vi "Sub_Online_FFT.vi"(9 "Bound to 1st Frequency":bool=TRUE, 10 "Frequency Method":T4(ring), 11 "Experiment in":T1) -> (3 "Experiment out":T2)   [LabVIEW 2021]
uses:
  Control 1.ctl
  <vilib>/Analysis/4window.llb/Hanning Window (DBL).vi
  <vilib>/Analysis/5stat.llb/RMS (DBL).vi
  <vilib>/Analysis/4window.llb/Hamming Window (DBL).vi
  <vilib>/Analysis/2dsp.llb/Real FFT.vi
  <vilib>/Analysis/4window.llb/AllCosWindow (DBL).vi
  <vilib>/addons/Time Series Analysis/Series Preprocess.llb/TSA Moving Average (Array).vi
  <vilib>/Analysis/NI_AALPro.lvlib
  <vilib>/addons/_Advanced Signal Processing/NI_AdvSigProcTSA.lvlib
panel:
  in  "Frequency selection method":T3(ring)
  in  "Use Top N freq components":i32=5 min=1 max=50 step=1
  out "Low-Energy Warning":bool
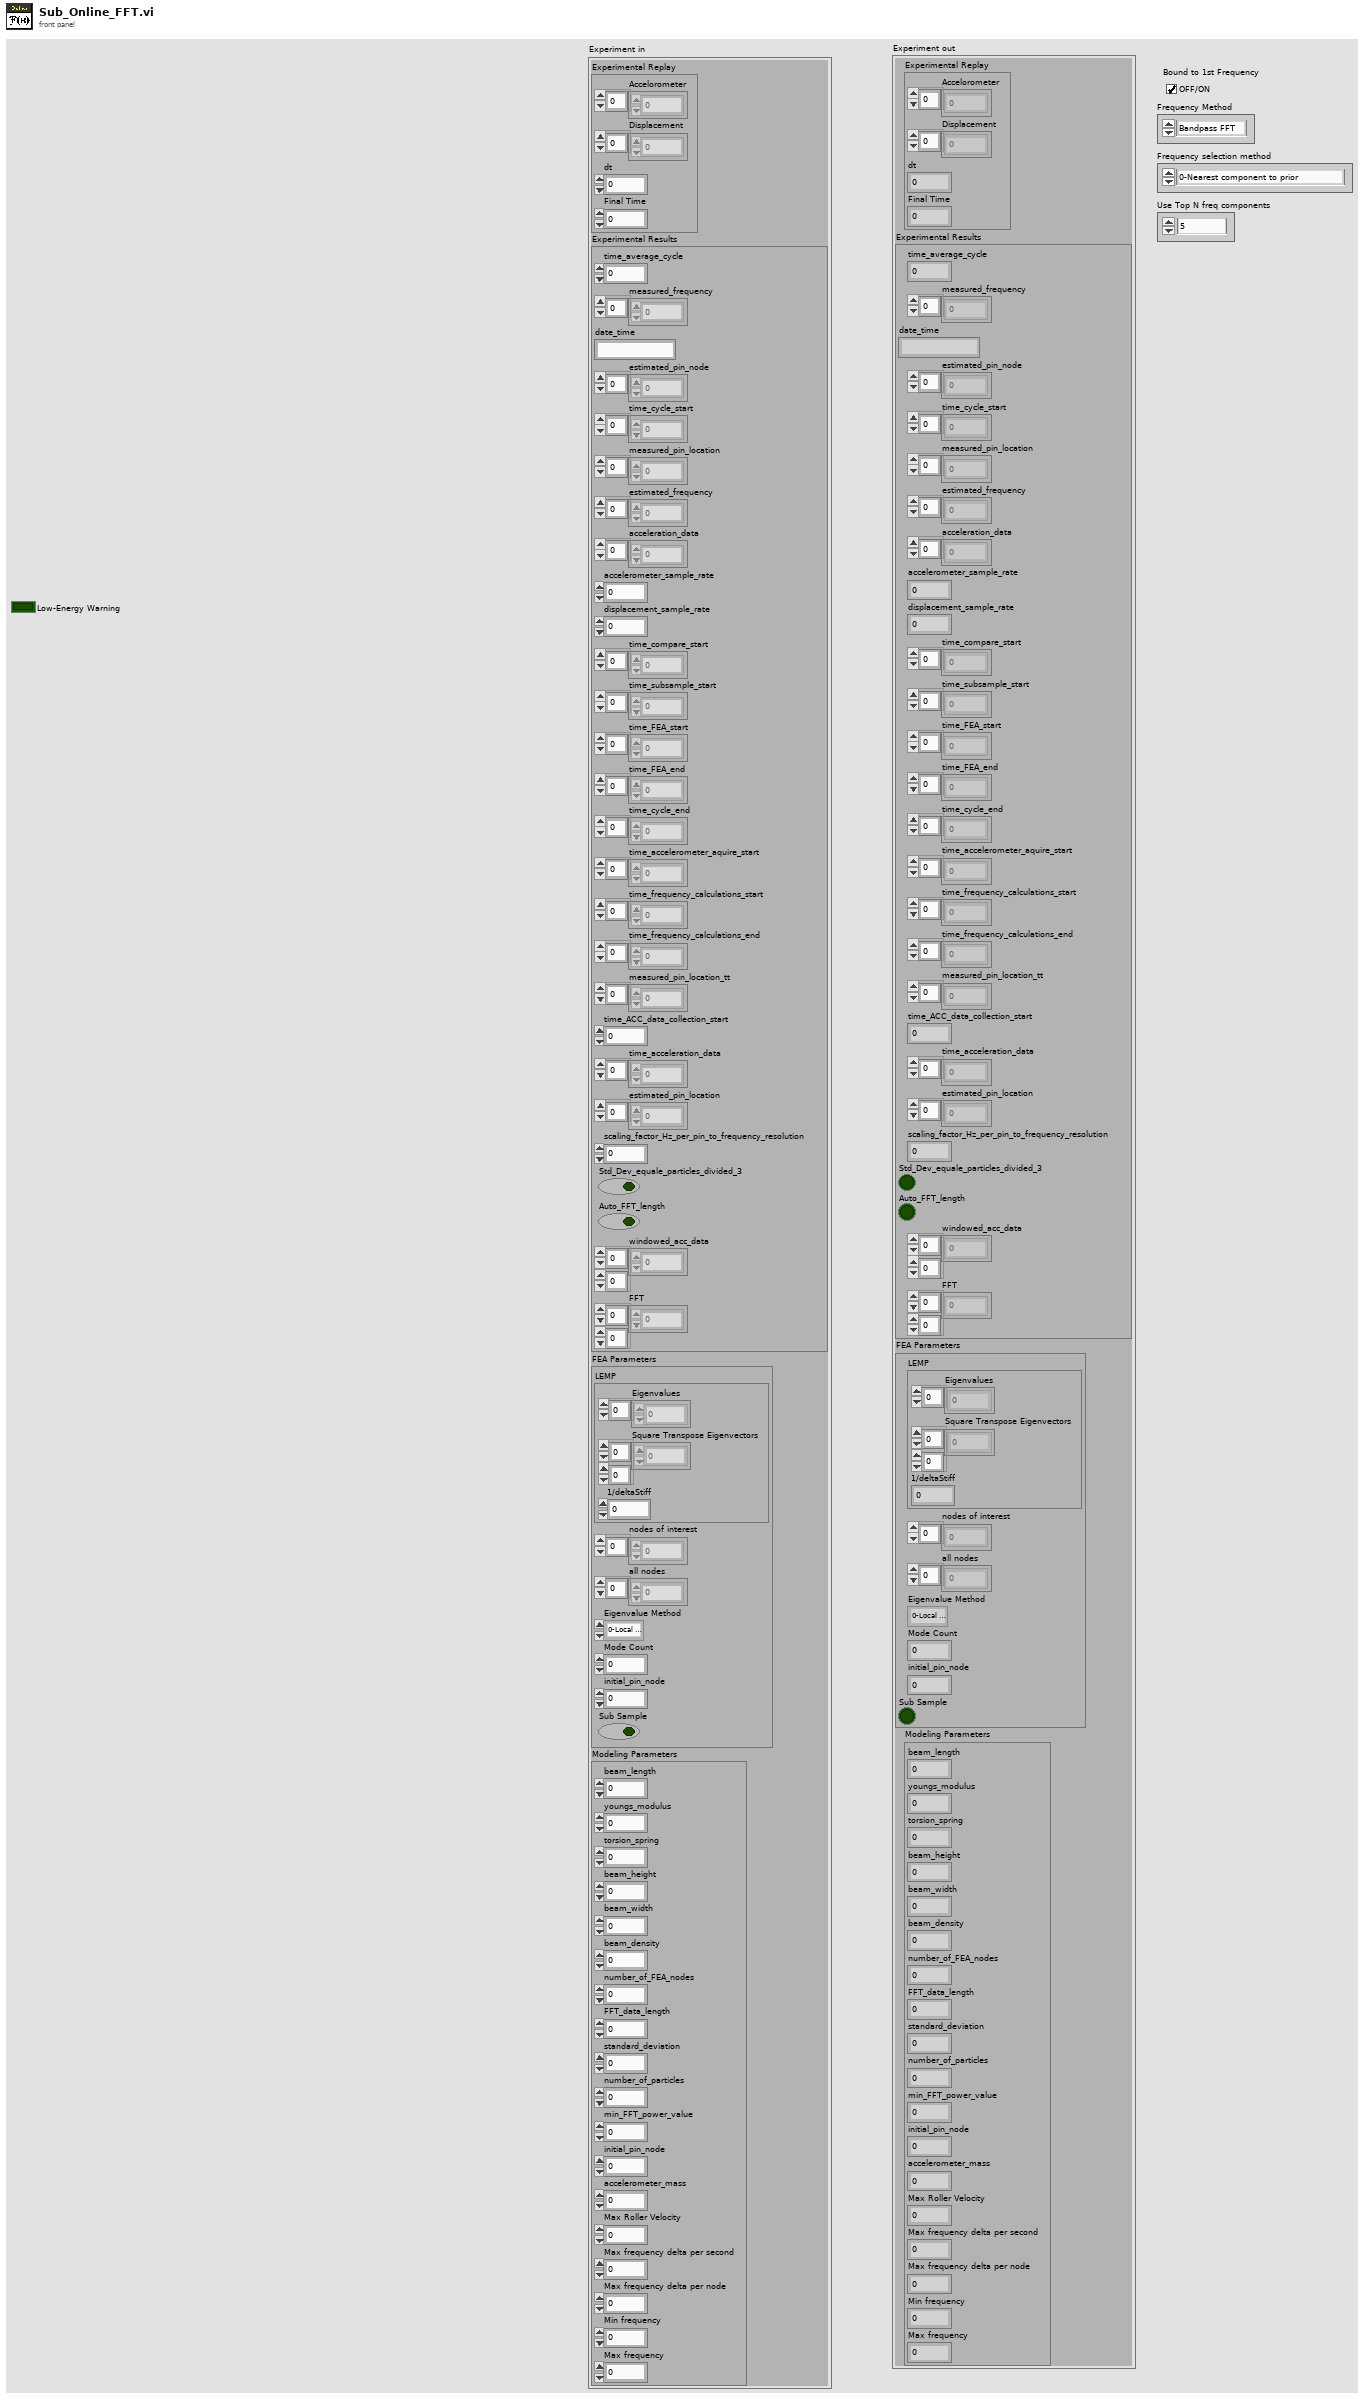
[diagram p1: front panel]
types:
  T1 = cluster{"Experimental Replay":cluster{"Accelorometer":dbl[], "Displacement":dbl[], "dt":dbl, "Final Time":dbl}, "Experimental Results":cluster{"time_average_cycle":dbl, "measured_frequency":dbl[], "date_time":string, "estimated_pin_node":i32[], "time_cycle_start":dbl[], "measured_pin_location":dbl[], "estimated_frequency":dbl[], "acceleration_data":dbl[], "accelerometer_sample_rate":dbl, "displacement_sample_rate":dbl, "time_compare_start":dbl[], "time_subsample_start":dbl[], "time_FEA_start":dbl[], "time_FEA_end":dbl[], "time_cycle_end":dbl[], "time_accelerometer_aquire_start":dbl[], "time_frequency_calculations_start":dbl[], "time_frequency_calculations_end":dbl[], "measured_pin_location_tt":dbl[], "time_ACC_data_collection_start":dbl, "time_acceleration_data":dbl[], "estimated_pin_location":dbl[], "scaling_factor_Hz_per_pin_to_frequency_resolution":dbl, "Std_Dev_equale_particles_divided_3":bool, "Auto_FFT_length":bool, "windowed_acc_data":dbl[][], "FFT":dbl[][]}, "FEA Parameters":cluster{"LEMP":cluster{"Eigenvalues":dbl[], "Square Transpose Eigenvectors":dbl[][], "1/deltaStiff":dbl}, "nodes of interest":i32[], "all nodes":i32[], "Eigenvalue Method":enum16{"0-Local Eigen Modification Procedure", "1-LabVIEW generalized eigenvalues", "2-LabVIEW M^-1K eigenvalues", "3-LabVIEW Cholesky Factorization", "4-Cholesky Factorization CPU SGL", "5-Cholesky Factorization CPU FXP", "6-Cholesky Factorization FPGA SGL", "7-Cholesky Factorization FPGA SGL SCL"}, "Mode Count":i32, "initial_pin_node":i32, "Sub Sample":bool}, "Modeling Parameters":cluster{"beam_length":dbl, "youngs_modulus":dbl, "torsion_spring":dbl, "beam_height":dbl, "beam_width":dbl, "beam_density":dbl, "number_of_FEA_nodes":i32, "FFT_data_length":i32, "standard_deviation":dbl, "number_of_particles":i32, "min_FFT_power_value":dbl, "initial_pin_node":i32, "accelerometer_mass":dbl, "Max Roller Velocity":dbl, "Max frequency delta per second":dbl, "Max frequency delta per node":dbl, "Min frequency":dbl, "Max frequency":dbl}}
  T2 = typedef "Control 1.ctl" = cluster{"Experimental Replay":cluster{"Accelorometer":dbl[], "Displacement":dbl[], "dt":dbl, "Final Time":dbl}, "Experimental Results":cluster{"time_average_cycle":dbl, "measured_frequency":dbl[], "date_time":string, "estimated_pin_node":i32[], "time_cycle_start":dbl[], "measured_pin_location":dbl[], "estimated_frequency":dbl[], "acceleration_data":dbl[], "accelerometer_sample_rate":dbl, "displacement_sample_rate":dbl, "time_compare_start":dbl[], "time_subsample_start":dbl[], "time_FEA_start":dbl[], "time_FEA_end":dbl[], "time_cycle_end":dbl[], "time_accelerometer_aquire_start":dbl[], "time_frequency_calculations_start":dbl[], "time_frequency_calculations_end":dbl[], "measured_pin_location_tt":dbl[], "time_ACC_data_collection_start":dbl, "time_acceleration_data":dbl[], "estimated_pin_location":dbl[], "scaling_factor_Hz_per_pin_to_frequency_resolution":dbl, "Std_Dev_equale_particles_divided_3":bool, "Auto_FFT_length":bool, "windowed_acc_data":dbl[][], "FFT":dbl[][]}, "FEA Parameters":cluster{"LEMP":cluster{"Eigenvalues":dbl[], "Square Transpose Eigenvectors":dbl[][], "1/deltaStiff":dbl}, "nodes of interest":i32[], "all nodes":i32[], "Eigenvalue Method":enum16{"0-Local Eigen Modification Procedure", "1-LabVIEW generalized eigenvalues", "2-LabVIEW M^-1K eigenvalues", "3-LabVIEW Cholesky Factorization", "4-Cholesky Factorization CPU SGL", "5-Cholesky Factorization CPU FXP", "6-Cholesky Factorization FPGA SGL", "7-Cholesky Factorization FPGA SGL SCL"}, "Mode Count":i32, "initial_pin_node":i32, "Sub Sample":bool}, "Modeling Parameters":cluster{"beam_length":dbl, "youngs_modulus":dbl, "torsion_spring":dbl, "beam_height":dbl, "beam_width":dbl, "beam_density":dbl, "number_of_FEA_nodes":i32, "FFT_data_length":i32, "standard_deviation":dbl, "number_of_particles":i32, "min_FFT_power_value":dbl, "initial_pin_node":i32, "accelerometer_mass":dbl, "Max Roller Velocity":dbl, "Max frequency delta per second":dbl, "Max frequency delta per node":dbl, "Min frequency":dbl, "Max frequency":dbl}}
  T3 = enum16{"0-Nearest component to prior ", "1-Coerce maximum differential", "2-Average with nearest component", "3-Top by power", "4-Lowest major component", "5-Average with lowest component"}
  T4 = enum16{"Bandpass FFT", "Tone", "FFT", "Custom Filter"}
  T5 = cluster{"Accelorometer":dbl[], "Displacement":dbl[], "dt":dbl, "Final Time":dbl}
  T6 = cluster{"time_average_cycle":dbl, "measured_frequency":dbl[], "date_time":string, "estimated_pin_node":i32[], "time_cycle_start":dbl[], "measured_pin_location":dbl[], "estimated_frequency":dbl[], "acceleration_data":dbl[], "accelerometer_sample_rate":dbl, "displacement_sample_rate":dbl, "time_compare_start":dbl[], "time_subsample_start":dbl[], "time_FEA_start":dbl[], "time_FEA_end":dbl[], "time_cycle_end":dbl[], "time_accelerometer_aquire_start":dbl[], "time_frequency_calculations_start":dbl[], "time_frequency_calculations_end":dbl[], "measured_pin_location_tt":dbl[], "time_ACC_data_collection_start":dbl, "time_acceleration_data":dbl[], "estimated_pin_location":dbl[], "scaling_factor_Hz_per_pin_to_frequency_resolution":dbl, "Std_Dev_equale_particles_divided_3":bool, "Auto_FFT_length":bool, "windowed_acc_data":dbl[][], "FFT":dbl[][]}
  T7 = cluster{"beam_length":dbl, "youngs_modulus":dbl, "torsion_spring":dbl, "beam_height":dbl, "beam_width":dbl, "beam_density":dbl, "number_of_FEA_nodes":i32, "FFT_data_length":i32, "standard_deviation":dbl, "number_of_particles":i32, "min_FFT_power_value":dbl, "initial_pin_node":i32, "accelerometer_mass":dbl, "Max Roller Velocity":dbl, "Max frequency delta per second":dbl, "Max frequency delta per node":dbl, "Min frequency":dbl, "Max frequency":dbl}
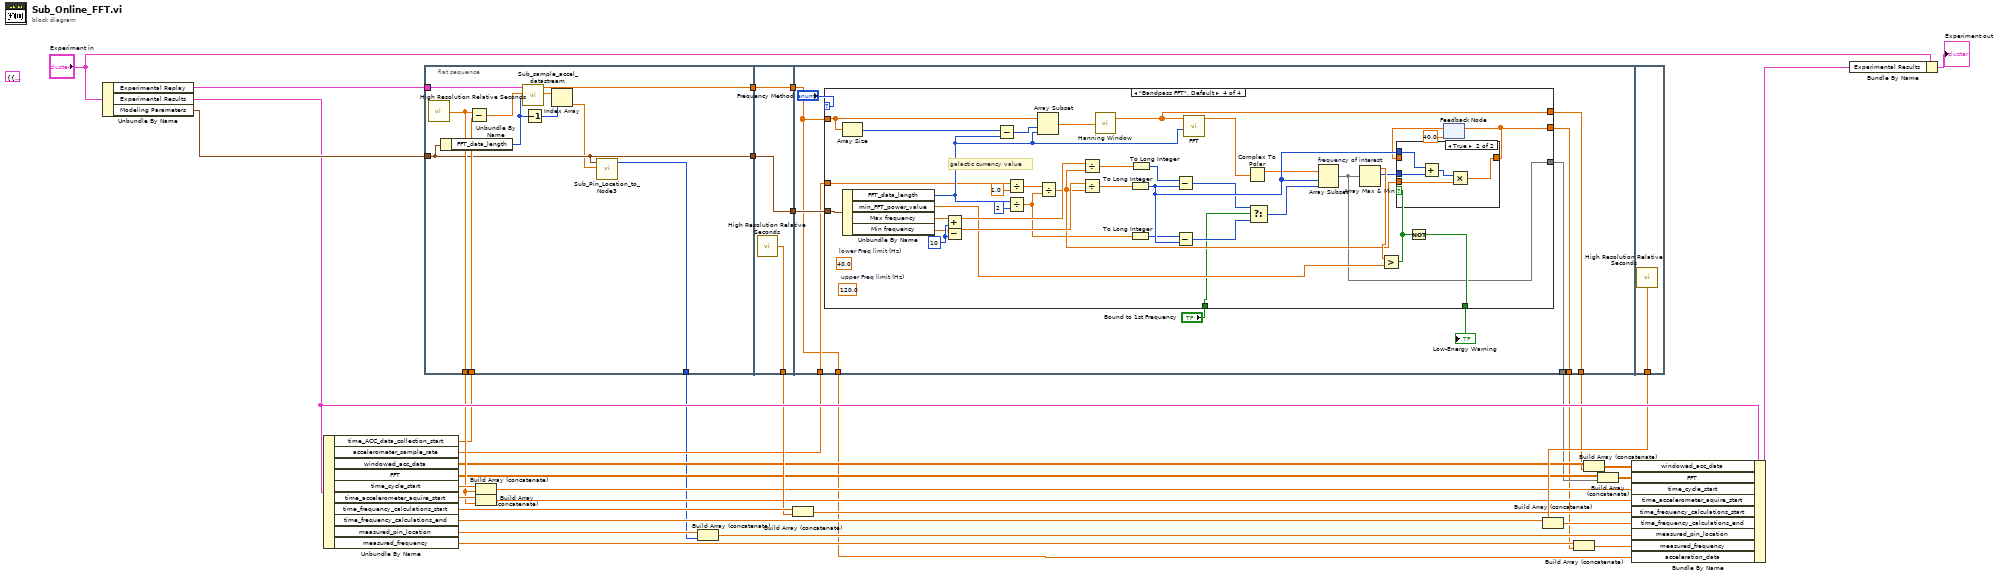
[diagram p0: block diagram]
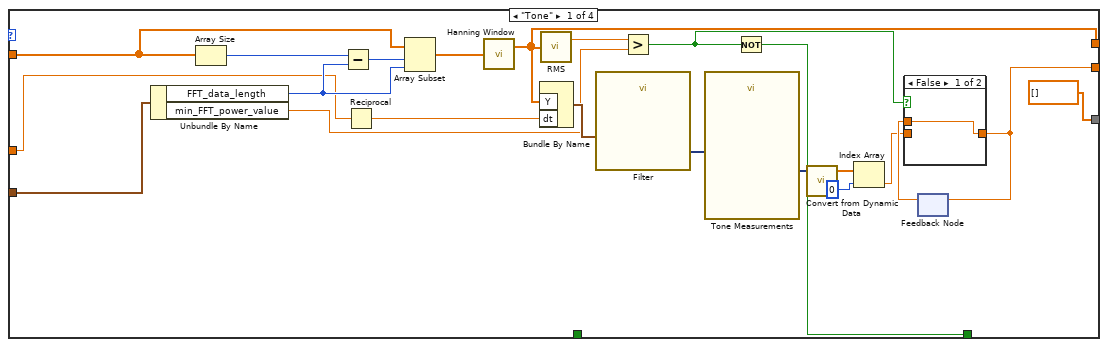
[diagram p2: hidden frame]
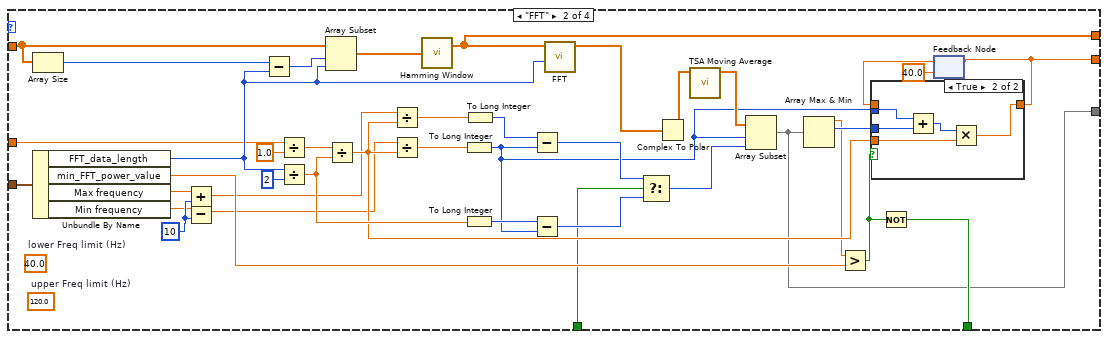
[diagram p4: hidden frame]
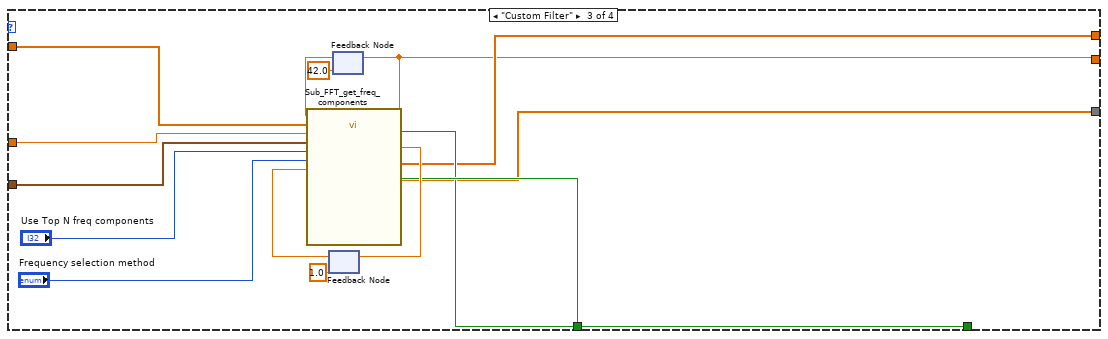
[diagram p6: hidden frame]
diagram:
  (unwired) T1 {"Experimental Replay"={"Accelorometer"=[], "Displacement"=[], "dt"=0.0, "Final Time"=0.0}, "Experimental Results"={"time_average_cycle"=0.0, "measured_frequency"=[], "date_time"="", "estimated_pin_node"=[], "time_cycle_start"=[], "measured_pin_location"=[], "estimated_frequency"=[], "acceleration_data"=[], "accelerometer_sample_rate"=0.0, "displacement_sample_rate"=0.0, "time_compare_start"=[], "time_subsample_start"=[], "time_FEA_start"=[], "time_FEA_end"=[], "time_cycle_end"=[], "time_accelerometer_aquire_start"=[], "time_frequency_calculations_start"=[], "time_frequency_calculations_end"=[], "measured_pin_location_tt"=[], "time_ACC_data_collection_start"=0.0, "time_acceleration_data"=[], "estimated_pin_location"=[], "scaling_factor_Hz_per_pin_to_frequency_resolution"=0.0, "Std_Dev_equale_particles_divided_3"=FALSE, "Auto_FFT_length"=FALSE, "windowed_acc_data"=[], "FFT"=[]}, "FEA Parameters"={"LEMP"={"Eigenvalues"=[], "Square Transpose Eigenvectors"=[], "1/deltaStiff"=0.0}, "nodes of interest"=[], "all nodes"=[], "Eigenvalue Method"=enum."0-Local Eigen Modification Procedure", "Mode Count"=0, "initial_pin_node"=0, "Sub Sample"=FALSE}, "Modeling Parameters"={"beam_length"=0.0, "youngs_modulus"=0.0, "torsion_spring"=0.0, "beam_height"=0.0, "beam_width"=0.0, "beam_density"=0.0, "number_of_FEA_nodes"=0, "FFT_data_length"=0, "standard_deviation"=0.0, "number_of_particles"=0, "min_FFT_power_value"=0.0, "initial_pin_node"=0, "accelerometer_mass"=0.0, "Max Roller Velocity"=0.0, "Max frequency delta per second"=0.0, "Max frequency delta per node"=0.0, "Min frequency"=0.0, "Max frequency"=0.0}} ("Experiment")
  n1 = Unbundle By Name("Experiment in") -> ("Experimental Replay"=w36:T5, "Experimental Results"=w27:T6, "Modeling Parameters"=w35:T7)
  n2 = Unbundle By Name(w27) -> ("time_ACC_data_collection_start"=w11:dbl, "accelerometer_sample_rate"=w10:dbl, "windowed_acc_data"=w9:dbl[][], "FFT"=w7:dbl[][], "time_cycle_start"=w18:dbl[], "time_accelerometer_aquire_start"=w17:dbl[], "time_frequency_calculations_start"=w21:dbl[], "time_frequency_calculations_end"=w26:dbl[], "measured_pin_location"=w19:dbl[], "measured_frequency"=w24:dbl[])
  n3 = flat-sequence {
    tunnel: w35 -> [w39]
    tunnel: [w43] -> w34
    tunnel: [w39] -> w32
    tunnel: [w47] -> w16
    tunnel: [w37] -> w2
    tunnel: w11 -> [w46]
    tunnel: w36 -> [w44]
    tunnel: w34 -> [w50]
    tunnel: [w50] -> w33
    tunnel: w32 -> [w49]
    tunnel: [w49] -> w31
    tunnel: [w48] -> w20
    tunnel: w33 -> [w51]
    tunnel: w31 -> [w58]
    tunnel: w10 -> [w55]
    tunnel: [w54] -> w4
    tunnel: [w53] -> w5
    tunnel: [w52] -> w3
    tunnel: [w51] -> w1
    tunnel: [w188] -> w25
    frame #0 {
      n4 = call <vilib>:"High Resolution Relative Seconds.vi"() -> ("relative seconds"=w47:dbl)
      n5 = Unbundle By Name(w39) -> ("FFT_data_length"=w40:i32)
      n6 = Subtract(x=w47, y=w46) -> (x-y=w45:dbl)
      n7 = call "Sub_sample_accel_datastream.vi"("FFT data length"=w40, "Simulation Time"=w45, "Experimental Replay"=w44) -> ("Displacment sample"=w42:dbl[], "Accelerometer sample"=w43:dbl[])  [unwired: 7 in]
      n8 = Decrement(x=w40) -> (x-1=w41:i32)
      n9 = Index Array(array=w42, index=w41) -> (element=w38:dbl)
      n10 = call "Sub_Pin_Location_to_Node3.vi"("Pin Location"=w38, "Modeling Parameters"=w39) -> ("DOF of Interest"=w37:i32)  [unwired: 9 in]
    }
    frame #1 {
      n11 = call <vilib>:"High Resolution Relative Seconds.vi"() -> ("relative seconds"=w48:dbl)
    }
    frame #2 {
      n12 = case shown="\"Bandpass FFT\", Default" "Frequency Method" {
        tunnel: [w69 w98 w132 w152] -> w52
        tunnel: [w71 w101 w135 w147] -> w54
        tunnel: w51 -> [w73 w104 w138 w155]
        tunnel: [w66 w100 w136 w154] -> w59
        tunnel: w58 -> [w64 w103 w139 w156]
        tunnel: "Bound to 1st Frequency" -> [_ w102 w140 w153]
        tunnel: [dbl[] [] ("Real freq comp (out)") w93 w130 w149] -> w53
        tunnel: w55 -> [w60 w84 w129 w144]
        frame "Tone" {
          n13 = Unbundle By Name(w64) -> ("FFT_data_length"=w62:i32, "min_FFT_power_value"=w63:dbl)
          n14 = Array Size(array=w73) -> (size(s)=w81:i32)
          n15 = Subtract(x=w81, y=w62) -> (x-y=w80:i32)
          n16 = Reciprocal(x=w60) -> (1/x=w65:dbl)
          n17 = Array Subset(array=w73, index=w80, length=w62) -> (w74:dbl[])
          n18 = call-poly <vilib>:"Hanning Window.vi"("X"=w74) -> ("Windowed X"=w71:dbl[])  [unwired: 1 out]
          n19 = Bundle By Name("Y"=w71, "dt"=w65) -> (w75:waveform(dbl))  [unwired: 1 in]
          n20 = call-poly <vilib>:"RMS.vi"("X"=w71) -> ("rms value"=w67:dbl)  [unwired: 1 out]
          n21 = call "Filter"("Signal"=w75) -> ("Filtered Signal"=w76:dynamicdata)  [unwired: 9 in, 1 out]
          n22 = Greater?(x=w67, y=w63) -> (0:w68:bool)
          n23 = call "Tone Measurements"("Signals"=w76) -> ("Frequency"=w77:dynamicdata)  [unwired: 9 in, 1 out]
          n24 = Not(x=w68) -> (.not. x?=w66:bool)
          n25 = call "Convert from Dynamic Data"("Dynamic Data Type"=w77) -> ("Array"=w78:dbl[])  [unwired: 3 in]
          n26 = Index Array(array=w78, index=0) -> (element=w70:dbl)
          n27 = feedback #1() -> (w72:dbl)  [unwired: 1 in]
          n28 = case shown="False" w68 {
            tunnel: [w82 w83] -> w69
            tunnel: w72 -> [w82 _]
            tunnel: w70 -> [_ w83]
            frame False {
            }
            frame True {
            }
          }
          n29 = feedback-in #1(w69) -> ()
        }
        frame "FFT" {
          w89 = 10
          (unwired) 120.0  # upper Freq limit (Hz)
          (unwired) 40.0  # lower Freq limit (Hz)
          n30 = Array Size(array=w104) -> (size(s)=w115:i32)
          n31 = Unbundle By Name(w103) -> ("FFT_data_length"=w88:i32, "min_FFT_power_value"=w105:dbl, "Max frequency"=w85:dbl, "Min frequency"=w86:dbl)
          n32 = Add(x=w85, y=w89) -> (x+y=w90:dbl)
          n33 = Subtract(x=w86, y=w89) -> (x-y=w91:dbl)
          n34 = Subtract(x=w115, y=w88) -> (x-y=w114:i32)
          n35 = Divide(x=w84, y=1.0) -> (x/y=w117:dbl)
          n36 = Divide(x=w88, y=2) -> (x/y=w116:dbl)
          n37 = Array Subset(array=w104, index=w114, length=w88) -> (w113:dbl[])
          n38 = Divide(x=w117, y=w116) -> (x/y=w111:dbl)
          n39 = Divide(x=w90, y=w111) -> (x/y=w110:dbl)
          n40 = Divide(x=w91, y=w111) -> (x/y=w121:dbl)
          n41 = call-poly <vilib>:"Hamming Window.vi"("X"=w113) -> ("Windowed X"=w101:dbl[])  [unwired: 1 out]
          n42 = To Long Integer(number=w121) -> (32bit integer=w92:i32)
          n43 = To Long Integer(number=w116) -> (32bit integer=w119:i32)
          n44 = To Long Integer(number=w110) -> (32bit integer=w109:i32)
          n45 = Subtract(x=w109, y=w92) -> (x-y=w107:i32)
          n46 = Subtract(x=w119, y=w92) -> (x-y=w106:i32)
          n47 = call-poly <vilib>:"FFT.vi"("FFT size"=w88, "X"=w101) -> ("FFT {X}"=w99:cdb[])  [unwired: 8 in, 1 out]
          n48 = Select(t=w107, s=w102, f=w106) -> (s? t:f=w108:i32)
          n49 = Complex To Polar(r * e^(i*theta)=w99) -> (r=w95:dbl[])  [unwired: 1 out]
          n50 = call-poly <vilib>:"TSA Moving Average.vi"("Xt"=w95) -> ("Xt out"=w94:dbl[])  [unwired: 9 in, 1 out]
          n51 = Array Subset(array=w94, index=w92, length=w108) -> (w93:dbl[])
          n52 = Array Max & Min(array=w93) -> (max value=w87:dbl, max index (indices)=w120:i32)  [unwired: 2 out]
          n53 = Greater?(x=w87, y=w105) -> (0:w112:bool)
          n54 = Not(x=w112) -> (.not. x?=w100:bool)
          n55 = feedback #2(40.0) -> (w97:dbl)
          n56 = case shown="True" w112 {
            tunnel: w120 -> [_ w124]
            tunnel: w92 -> [_ w125]
            tunnel: w111 -> [_ w126]
            tunnel: [w123 w127] -> w98
            tunnel: w97 -> [w123 _]
            frame False {
            }
            frame True {
              n57 = Add(x=w125, y=w124) -> (x+y=w128:i32)
              n58 = Multiply(x=w128, y=w126) -> (x*y=w127:dbl)
            }
          }
          n59 = feedback-in #2(w98) -> ()
        }
        frame "Custom Filter" {
          n60 = feedback #3(1.0 ("Slop factor (Feed back)")) -> (w142:dbl)
          n61 = feedback #4(42.0) -> (w141:dbl)
          n62 = call "Sub_FFT_get_freq_components.vi"("Prior Frequency Estimate (Feed forward)"=w141, "ACC Signal"=w138, "accelerometer_sample_rate"=w129, "Modeling Parameters"=w139, "Use Top N freq components"="Use Top N freq components", "Frequency selection method"="Frequency selection method", "Slop factor (Feed forward)"=w142, "Bound to 1st Frequency"=w140) -> ("Windowed X (out)"=w135:dbl[], "Real freq comp (out)"=w130:dbl[], "Next Frequency Estimate"=w132:dbl, "Low Energy"=w136:bool, "Slop factor (Feed back)"=w143:dbl)  [unwired: 15 in]
          n63 = feedback-in #3(w143) -> ()
          n64 = feedback-in #4(w132) -> ()
        }
        frame "Bandpass FFT", Default {
          w157 = 10
          (unwired) 120.0  # upper Freq limit (Hz)
          (unwired) 40.0  # lower Freq limit (Hz)
          # "galactic currency value"
          n65 = Array Size(array=w155) -> (size(s)=w166:i32)
          n66 = Unbundle By Name(w156) -> ("FFT_data_length"=w180:i32, "min_FFT_power_value"=w175:dbl, "Max frequency"=w145:dbl, "Min frequency"=w146:dbl)
          n67 = Add(x=w145, y=w157) -> (x+y=w179:dbl)
          n68 = Subtract(x=w146, y=w157) -> (x-y=w178:dbl)
          n69 = Subtract(x=w166, y=w180) -> (x-y=w167:i32)
          n70 = Divide(x=w144, y=1.0) -> (x/y=w164:dbl)
          n71 = Divide(x=w180, y=2) -> (x/y=w165:dbl)
          n72 = Array Subset(array=w155, index=w167, length=w180) -> (w148:dbl[])
          n73 = Divide(x=w164, y=w165) -> (x/y=w169:dbl)
          n74 = Divide(x=w179, y=w169) -> (x/y=w170:dbl)
          n75 = Divide(x=w178, y=w169) -> (x/y=w161:dbl)
          n76 = call-poly <vilib>:"Hanning Window.vi"("X"=w148) -> ("Windowed X"=w147:dbl[])  [unwired: 1 out]
          n77 = To Long Integer(number=w161) -> (32bit integer=w177:i32)
          n78 = To Long Integer(number=w165) -> (32bit integer=w163:i32)
          n79 = To Long Integer(number=w170) -> (32bit integer=w171:i32)
          n80 = Subtract(x=w171, y=w177) -> (x-y=w173:i32)
          n81 = Subtract(x=w163, y=w177) -> (x-y=w174:i32)
          n82 = call-poly <vilib>:"FFT.vi"("FFT size"=w180, "X"=w147) -> ("FFT {X}"=w151:cdb[])  [unwired: 8 in, 1 out]
          n83 = Complex To Polar(r * e^(i*theta)=w151) -> (r=w150:dbl[])  [unwired: 1 out]
          n84 = Select(t=w173, s=w153, f=w174) -> (s? t:f=w172:i32)
          n85 = Array Subset "frequency of interest"(array=w150, index=w177, length=w172) -> (w149:dbl[])
          n86 = Array Max & Min(array=w149) -> (max value=w181:dbl, max index (indices)=w162:i32)  [unwired: 2 out]
          n87 = Greater?(x=w181, y=w175) -> (0:w168:bool)
          n88 = Not(x=w168) -> (.not. x?=w154:bool)
          n89 = feedback #5(40.0) -> (w176:dbl)
          n90 = case shown="True" w168 {
            tunnel: w162 -> [_ w183]
            tunnel: w177 -> [_ w184]
            tunnel: w169 -> [_ w185]
            tunnel: [w182 w186] -> w152
            tunnel: w176 -> [w182 _]
            frame False {
            }
            frame True {
              n91 = Add(x=w184, y=w183) -> (x+y=w187:i32)
              n92 = Multiply(x=w187, y=w185) -> (x*y=w186:dbl)
            }
          }
          n93 = feedback-in #5(w152) -> ()
        }
      }
      "Low-Energy Warning" <- w59
    }
    frame #3 {
      n94 = call <vilib>:"High Resolution Relative Seconds.vi"() -> ("relative seconds"=w188:dbl)
    }
  }
  n95 = Build Array (concatenate)(w18, w16) -> (w14:dbl[])
  n96 = Build Array (concatenate)(w17, w16) -> (w13:dbl[])
  n97 = Build Array (concatenate)(w19, w2) -> (w15:dbl[])
  n98 = Build Array (concatenate)(w21, w20) -> (w12:dbl[])
  n99 = Build Array (concatenate)(w26, w25) -> (w22:dbl[])
  n100 = Build Array (concatenate)(w24, w3) -> (w23:dbl[])
  n101 = Build Array (concatenate)(w9, w4) -> (w8:dbl[][])
  n102 = Build Array (concatenate)(w7, w5) -> (w6:dbl[][])
  n103 = Bundle By Name(cluster=w27, "windowed_acc_data"=w8, "FFT"=w6, "time_cycle_start"=w14, "time_accelerometer_aquire_start"=w13, "time_frequency_calculations_start"=w12, "time_frequency_calculations_end"=w22, "measured_pin_location"=w15, "measured_frequency"=w23, "acceleration_data"=w1) -> (w28:T6)
  n104 = Bundle By Name(cluster="Experiment in", "Experimental Results"=w28) -> (→"Experiment out":T1)
